vi "PLC.Dial800.OPC Disconnect.vi"(8 "error in (no error)":errorcluster, 9 "ms timeout (1000)":i32=100, 11 "Var URLs In":T1[](array[typedef])) -> (0 "error out":errorcluster)   [LabVIEW 2018]
uses:
  PLC.Dial800.Var URL Item.ctl
  PLC.Dial800.VarNameSelector.ctl
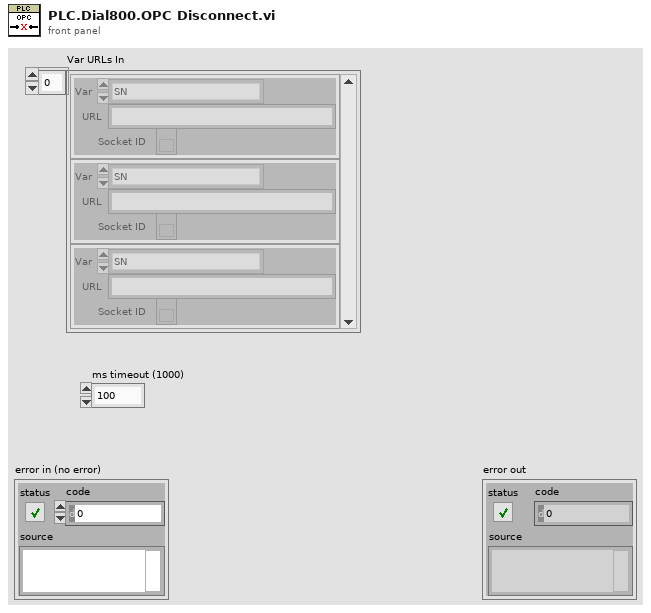
[diagram p1: front panel]
types:
  T1 = typedef "PLC.Dial800.Var URL Item.ctl" = cluster{"Var":T2, "URL":string, "Socket ID":refnum<k13>}
  T2 = typedef "PLC.Dial800.VarNameSelector.ctl" = enum16{"SN", "Reset", "HeartBeat_PLC", "Heartbeat_PC", "Start", "Running", "Done", "Pass"}
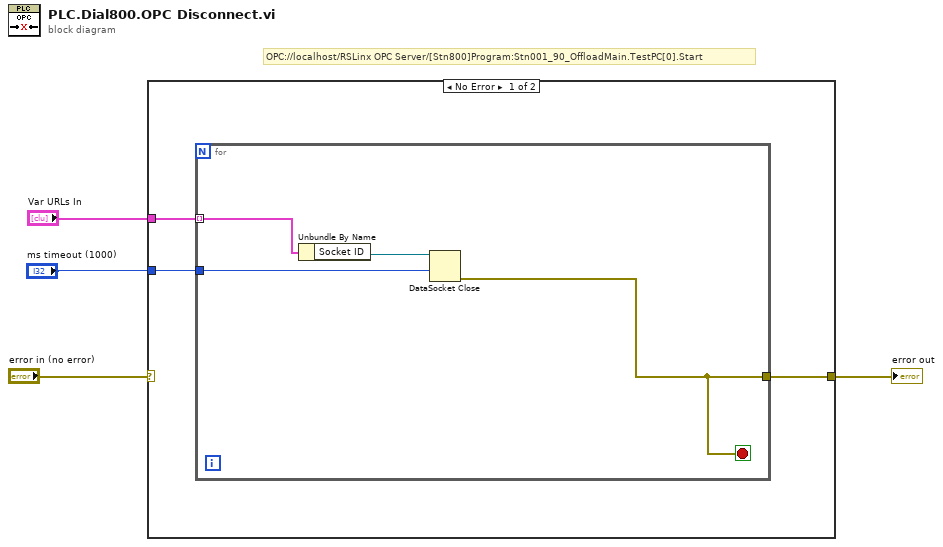
[diagram p0: block diagram]
diagram:
  # "OPC://localhost/RSLinx OPC Server/[Stn800]Program:Stn001_90_OffloadMain.TestPC[0].Start"
  n1 = case shown="No Error" "error in (no error)" {
    selector: "error in (no error)" -> [_ w12]
    tunnel: [w7 w12] -> w3
    tunnel: "Var URLs In" -> [w6 _]
    tunnel: "ms timeout (1000)" -> [w5 _]
    frame No Error {
      n2 = for {
        tunnel: [w8] -> w7
        tunnel: w6 -> [w9] mode=indexing
        tunnel: w5 -> [w11]
        stop <- w8 stop-if-true
        n3 = Unbundle By Name(w9) -> ("Socket ID"=w10:refnum<k13>)
        n4 = DataSocket Close(9:w11, 11:w10) -> (0:w8:errorcluster)  [unwired: 1 in, 1 out]
      }
    }
    frame Error {
    }
  }
  "error out" <- w3
